vi "LoadSequenceString.vi"(0 "Sequence String":string) -> (1 "Chapter":string="Chapter(DopplerCooling,\n10100000 00000000 00000000)\nChapter(Pump,\n01000000 00000000 00000000)\nChapter(Pulsed,\n00100000 00000000 00000000,\n00000100 00000000 00000000,\n00000000 10000000 00000000,\n01000000 00000000 01000000)\nChapter(Zero,\n00000000 00000000 00000000)\nChapter(One,\n11111111 11111111 11111111)\nZero(1)\nOne(1)\nZero(1)\nOne(1)\nZero(1)\nOne(1)\nZero(1)\nOne(1)\nZero(1)\nOne(1)\n", 2 "Sequence":string)   [LabVIEW 2014]
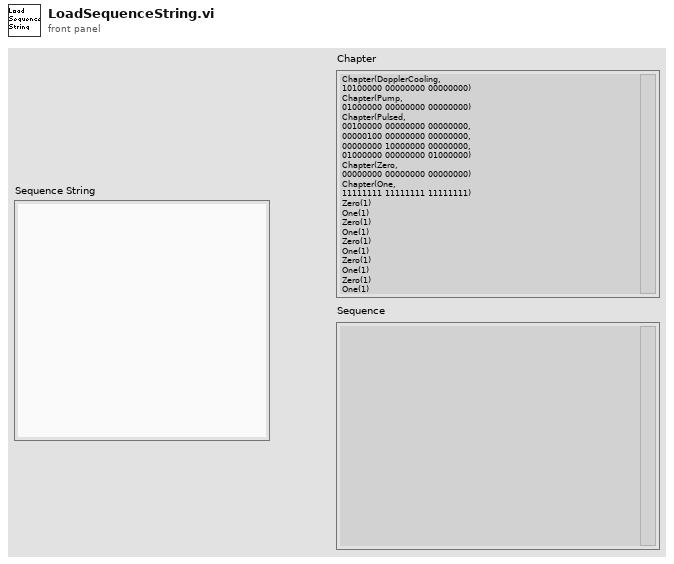
[diagram p1: front panel]
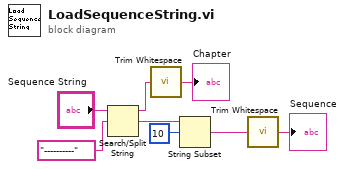
[diagram p0: block diagram]
diagram:
  n1 = Search/Split String(string="Sequence String", search string/char (-)="----------") -> (substring before match=w4:string, match + rest of string=w8:string)  [unwired: 1 in, 1 out]
  n2 = call <vilib>:"Trim Whitespace.vi"("string"=w4) -> ("trimmed string"=→"Chapter":string)  [unwired: 1 in]
  n3 = String Subset(string=w8, offset (0)=10) -> (substring=w5:string)  [unwired: 1 in]
  n4 = call <vilib>:"Trim Whitespace.vi"("string"=w5) -> ("trimmed string"=→"Sequence":string)  [unwired: 1 in]
